vi "setSerializedData.vi"(0 "reference":refnum<class "AbstractNode.lvclass">, 1 "parent":refnum<class "AbstractNode.lvclass">, 2 "children":refnum<class "AbstractNode.lvclass">[](array[class]), 3 "xmlOut":string, 5 "error in (no error)":errorcluster) -> (14 "reference out":refnum<class "AbstractNode.lvclass">, 19 "error out":errorcluster)   [LabVIEW 2020, in "AbstractNode.lvclass"]
doc: "Sets data that has been stored store"
uses:
  <resource>/Framework/Providers/Open_GDS/UML/AbstractNode_class/AbstractNode.lvclass
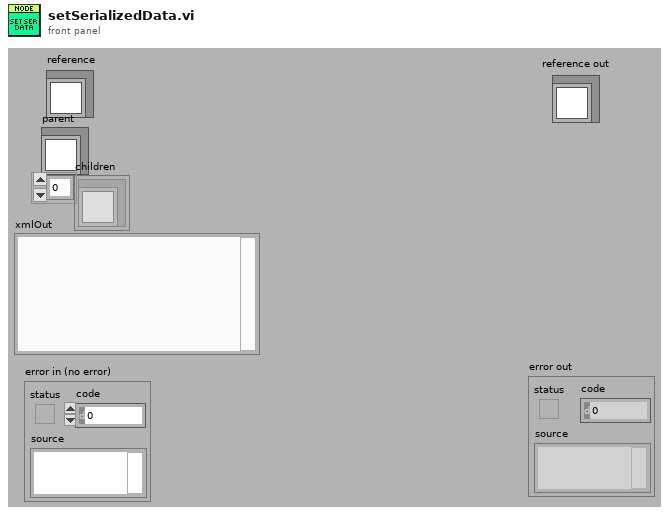
[diagram p1: front panel]
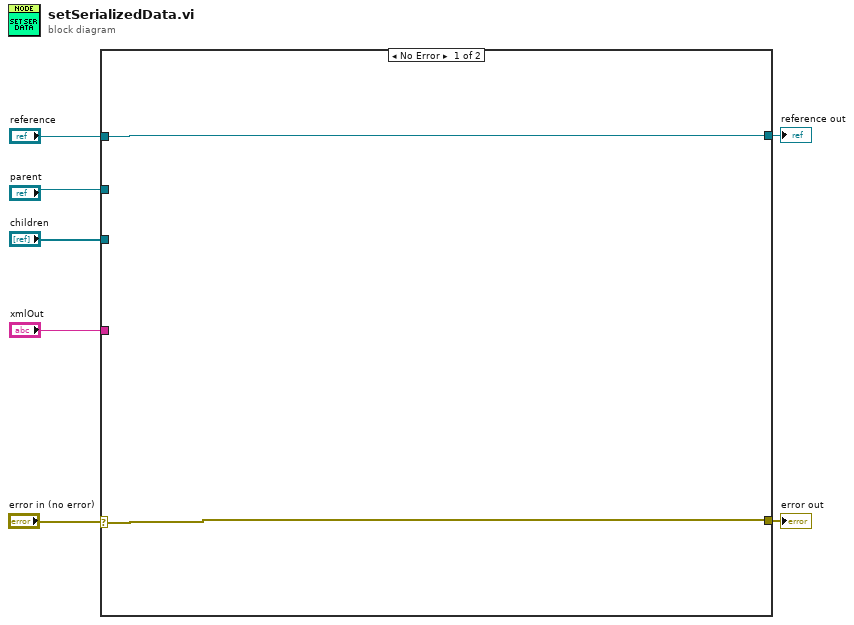
[diagram p0: block diagram]
diagram:
  n1 = case shown="No Error" "error in (no error)" {
    selector: "error in (no error)" -> [w8 w10]
    tunnel: "reference" -> [w9 w11]
    tunnel: [w8 w10] -> w6
    tunnel: [w9 w11] -> w5
    tunnel: "parent" -> [_ _]
    tunnel: "children" -> [_ _]
    tunnel: "xmlOut" -> [_ _]
    frame No Error {
    }
    frame Error {
    }
  }
  "reference out" <- w5
  "error out" <- w6
